vi "OA Enable Mode.vi"(11 "pcModeName":string) -> (3 "function return":u32)   [LabVIEW 2018, in "AndorSDK.lvlib"]
doc: "EXPNETTYPE unsigned int WINAPI OA_EnableMode(const char * const pcModeName);"
uses:
  AndorSDK.lvlib
  ATMCD32D.dll
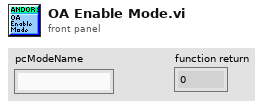
[diagram p1: front panel]
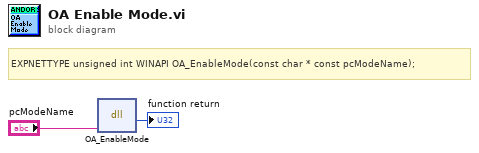
[diagram p0: block diagram]
diagram:
  # "EXPNETTYPE unsigned int WINAPI OA_EnableMode(const char * const pcModeName);"
  n1 = dll-call lib="PTH2babs E\nPersönliches02 - Arbeit03-HiwijobsLabviewCodelibANDOR\tAndor SDK\nATMCD32D.*" fn="OA_EnableMode"("pcModeName"="pcModeName") -> (→"function return":u32)  [unwired: 4 in, 2 out]
